vi "PID (Read).vi"(6 "ISOBUS address":T2=-1 caption="ISOBUS address (-1)", 8 "error in":errorcluster, 11 "Mercury Reference In":T4) -> (0 "error out":errorcluster, 2 "PID":T1 {"D" min=0.0 max=299.9 step=0.1 format="%#.1f"; "I" min=0.0 max=199.9 step=0.1 format="%#.1f"; "P" min=0.0 max=199.9 step=0.1 format="%#.1f"}, 3 "Mercury Reference Out":T4, 4 "Valid?":T3)   [LabVIEW 2016, in "Mercury iXX.lvlib" / "Control Loop.lvlib"]
doc: "Check the PID values of the PID associated with control loop."
uses:
  Control Loop.lvlib
  Controls/Mercury Reference.ctl
  Controls/Comms Transport Layer.ctl
  Private/Controls/Query Dynamic Reference.ctl
  Controls/Is Valid LED.ctl
  Controls/ISOBus Address.ctl
  Controls/PID cluster.ctl
  Private/Controls/Command Verbs.ctl
  Mercury iXX.lvlib
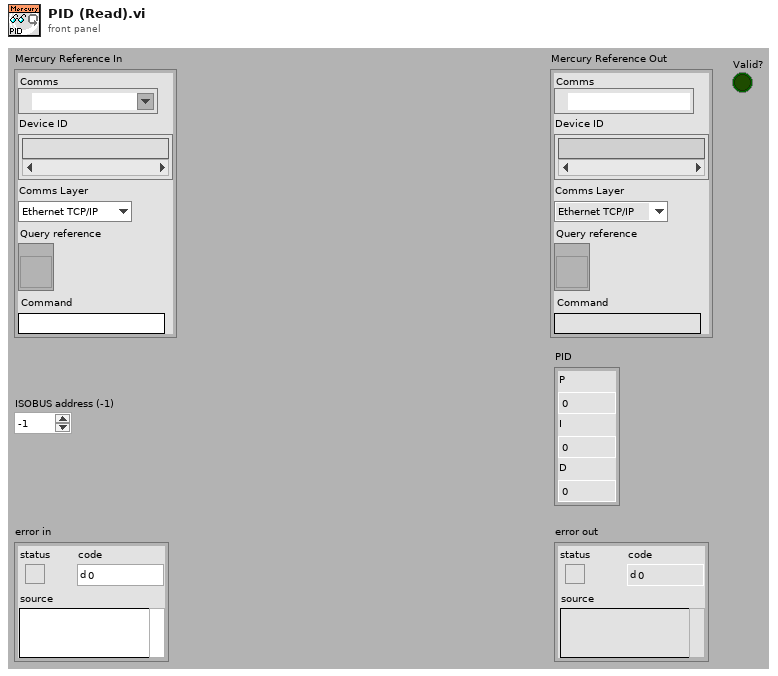
[diagram p1: front panel]
types:
  T1 = typedef "Mercury iXX.lvlib/Control Loop.lvlib/PID cluster.ctl" = cluster{"P":dbl, "I":dbl, "D":dbl}
  T2 = typedef "Mercury iXX.lvlib/ISOBus Address.ctl" = i32
  T3 = typedef "Mercury iXX.lvlib/Is Valid LED.ctl" = bool
  T4 = typedef "Mercury iXX.lvlib/Mercury Reference.ctl" = cluster{"Comms":refnum<visa-resource-name>, "Device ID":string[], "Comms Layer":T5, "Command":string, "Query reference":T6}
  T5 = typedef "Mercury iXX.lvlib/Comms Transport Layer.ctl" = enum16{"Ethernet TCP/IP", "USB", "ISOBus - RS-232", "GPIB"}
  T6 = typedef "Mercury iXX.lvlib/Query Dynamic Reference.ctl" = refnum<vi>
  T7 = typedef "Mercury iXX.lvlib/Command Verbs.ctl" = string
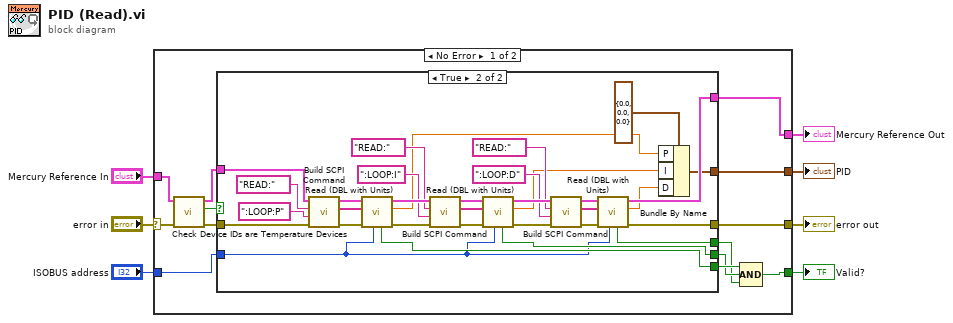
[diagram p0: block diagram]
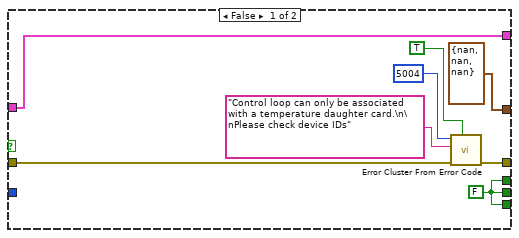
[diagram p2: hidden frame]
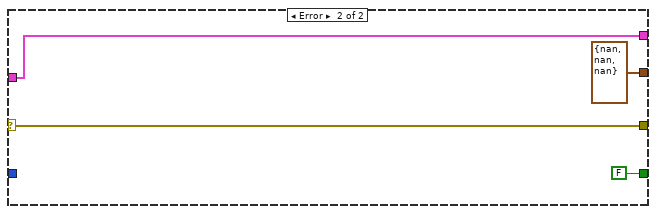
[diagram p3: hidden frame]
diagram:
  n1 = case shown="No Error" "error in" {
    selector: "error in" -> [w16 w63]
    tunnel: "Mercury Reference In" -> [w13 w64]
    tunnel: [w20 w64] -> w4
    tunnel: [w18 w63] -> w3
    tunnel: "ISOBUS address" -> [w19 _]
    tunnel: [w9 FALSE ("Valid?")] -> w2
    tunnel: [w8 T1 {"P"=nan, "I"=nan, "D"=nan} ("PID")] -> w1
    frame No Error {
      n2 = call "Check Device IDs are Temperature Devices.vi"("error in"=w16, "Mercury Reference In"=w13) -> ("error out"=w15:errorcluster, "Valid?"=w17:bool, "Mercury Reference Out"=w14:T4)  [unwired: 7 out]
      n3 = case shown="True" w17 {
        tunnel: w14 -> [w28 w41]
        tunnel: [w28 w38] -> w20
        tunnel: w15 -> [w26 w40]
        tunnel: w19 -> [_ w34]
        tunnel: [w27 w39] -> w18
        tunnel: [w22 w37] -> w12
        tunnel: [w22 w36] -> w11
        tunnel: [w22 w35] -> w10
        tunnel: [T1 {"P"=nan, "I"=nan, "D"=nan} ("PID") w29] -> w8
        frame False {
          w22 = T3 FALSE ("Valid?")
          n4 = call <vilib>:"Error Cluster From Error Code.vi"("show call chain? (False)"=TRUE, "error in (no error)"=w26, "error message (\"\")"="Control loop can only be associated with a temperature daughter card.\n\nPlease check device IDs" ("error message (\"\")"), "error code (0)"=5004) -> ("error out"=w27:errorcluster)  [unwired: 5 out]
        }
        frame True {
          n5 = call "Build SCPI Command.vi"("error in"=w40, "Noun(s)"=":LOOP:P" ("Command"), "Verb"=T7 "READ:", "Mercury Reference In"=w41) -> ("error out"=w42:errorcluster, "SCPI Message(s)"=w44:string[], "Mercury Reference Out"=w45:T4)  [unwired: 5 out]
          n6 = call "Read (DBL with Units).vi"("ISOBUS address"=w34, "error in"=w42, "SCPI Message(s)"=w44, "Mercury Reference In"=w45) -> ("error out"=w54:errorcluster, "Data (Dbl)"=w32:dbl, "Mercury Reference Out"=w59:T4, "Valid?"=w37:T3)  [unwired: 4 out]
          n7 = call "Build SCPI Command.vi"("error in"=w54, "Noun(s)"=":LOOP:I" ("Command"), "Verb"=T7 "READ:", "Mercury Reference In"=w59) -> ("error out"=w49:errorcluster, "SCPI Message(s)"=w47:string[], "Mercury Reference Out"=w46:T4)  [unwired: 5 out]
          n8 = call "Read (DBL with Units).vi"("ISOBUS address"=w34, "error in"=w49, "SCPI Message(s)"=w47, "Mercury Reference In"=w46) -> ("error out"=w55:errorcluster, "Data (Dbl)"=w31:dbl, "Mercury Reference Out"=w60:T4, "Valid?"=w36:T3)  [unwired: 4 out]
          n9 = call "Build SCPI Command.vi"("error in"=w55, "Noun(s)"=":LOOP:D" ("Command"), "Verb"=T7 "READ:", "Mercury Reference In"=w60) -> ("error out"=w50:errorcluster, "SCPI Message(s)"=w52:string[], "Mercury Reference Out"=w53:T4)  [unwired: 5 out]
          n10 = call "Read (DBL with Units).vi"("ISOBUS address"=w34, "error in"=w50, "SCPI Message(s)"=w52, "Mercury Reference In"=w53) -> ("error out"=w39:errorcluster, "Data (Dbl)"=w30:dbl, "Mercury Reference Out"=w38:T4, "Valid?"=w35:T3)  [unwired: 4 out]
          n11 = Bundle By Name(cluster=T1 {"P"=0.0, "I"=0.0, "D"=0.0} ("PID"), "P"=w32, "I"=w31, "D"=w30) -> (w29:T1)
        }
      }
      n12 = Compound Arithmetic op=AND(w12, w11, w10) -> (w9:T3)
    }
    frame Error {
    }
  }
  "Mercury Reference Out" <- w4
  "Valid?" <- w2
  "error out" <- w3
  "PID" <- w1
